vi "_076.vi"() -> ()   [LabVIEW 2024]
panel:
  out "index of element 2":i32
  out "index of element":i32
  # "Fundamentals :"
  # "5~>After running this VI,what is the value displayed in the o/p ?"
  # "Nrml Approach :"
  # "Dfrnt Approach :"
  # "( Work flow )"
  # "Search 1D-Array is used to get the particular element's index in that array . Starting index in search 1D-Array , The default val is zero. Suppose we have the same number in 2nd index and the 5th index but we have to find the 2nd same number means we have to give the starting index val & search , and we get the correct output.\nThe default val of the negative index & the undefined index is -1"
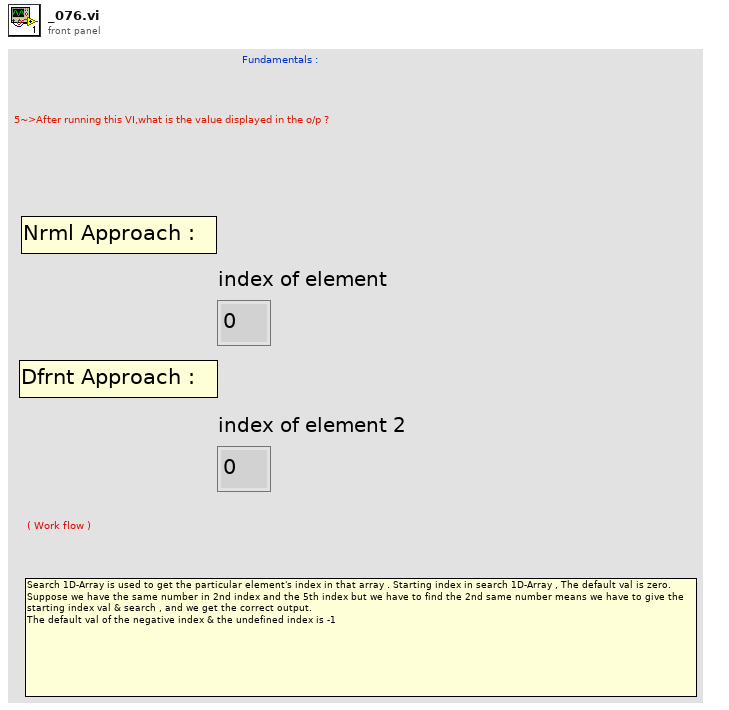
[diagram p1: front panel]
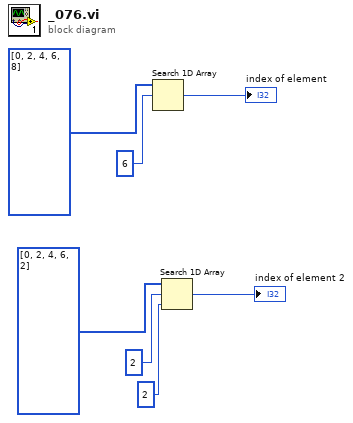
[diagram p0: block diagram]
diagram:
  n1 = Search 1D Array(1D array=i32[] [0, 2, 4, 6, 8], element=6) -> (index of element=→"index of element":i32)  [unwired: 1 in]
  n2 = Search 1D Array(1D array=i32[] [0, 2, 4, 6, 2], element=2, start index (0)=2) -> (index of element=→"index of element 2":i32)
